vi "LV SCISDK Detach Device.vi"(8 "error in (no error)":errorcluster, 10 "handle":u64, 11 "name":string) -> (0 "error out":errorcluster, 3 "function return":i32)   [LabVIEW 2021, in "SciSDK_Labview.lvlib"]
doc: "SCISDKLABVIEW_DLL_API int LV_SCISDK_DetachDevice(char* name, void* handle);"
uses:
  SciSDK_Labview.lvlib
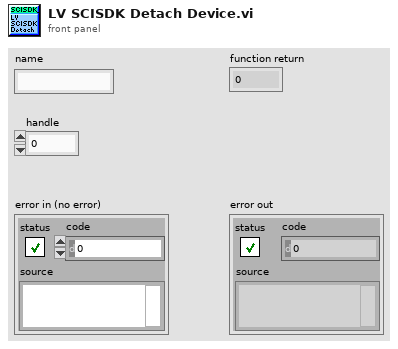
[diagram p1: front panel]
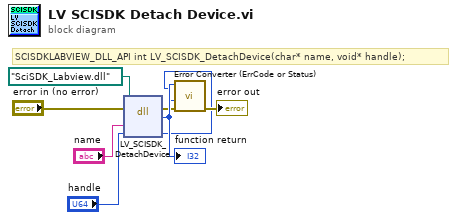
[diagram p0: block diagram]
diagram:
  # "SCISDKLABVIEW_DLL_API int LV_SCISDK_DetachDevice(char* name, void* handle);"
  n1 = dll-call lib="C:/git/scisdk/SciSDK_VC++/x64/Debug/SciSDK_Labview.dll" fn="LV_SCISDK_DetachDevice"(path in=path "SciSDK_Labview.dll", error in="error in (no error)", "name"="name", "handle"="handle") -> (error out=w4:errorcluster, "return type"=w8:i32, "handle"=w1:u64)  [unwired: 2 in, 1 out]
  "function return" <- w8
  n2 = call "Error Converter (ErrCode or Status).vi"("error in (no error)"=w4, "handle"=w1, "error code"=w8) -> ("error out"=→"error out":errorcluster)  [unwired: 8 in]
